vi "Format Data.vi"(0 "Potentiostat Galvanostat in":refnum<class "Potentiostat Galvanostat.lvclass">, 7 "Data Buffer":u32[][](array[numeric]), 11 "error in (no error)":errorcluster) -> (4 "Potentiostat Galvanostat out":refnum<class "Potentiostat Galvanostat.lvclass">, 8 "Data":sgl[][](array[numeric]), 15 "error out":errorcluster)   [LabVIEW 2018, in "Potentiostat Galvanostat.lvclass"]
doc: "The hardware conf object. The attribute “Conn” is the electrode\nconnection mode and the attribute “Ground” is the instrument\nground. See 5. Structures and Constants to have the value of these\nattributes."
uses:
  Potentiostat Galvanostat.lvclass
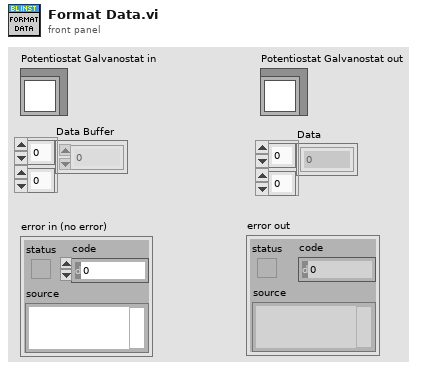
[diagram p1: front panel]
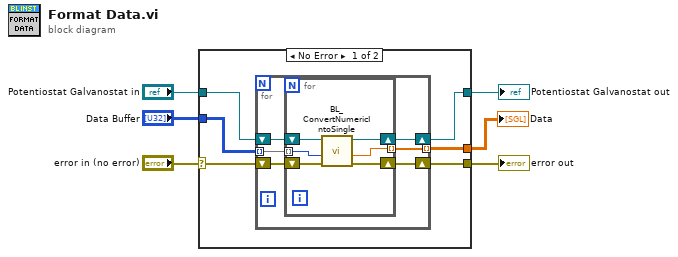
[diagram p0: block diagram]
diagram:
  n1 = case shown="No Error" "error in (no error)" {
    selector: "error in (no error)" -> [w8 w25]
    tunnel: "Data Buffer" -> [w7 _]
    tunnel: "Potentiostat Galvanostat in" -> [w12 w26]
    tunnel: [w11 _] -> w4
    tunnel: [w10 w25] -> w3
    tunnel: [w9 w26] -> w2
    frame No Error {
      n2 = for {
        tunnel: w7 -> [w18] mode=indexing
        tunnel: [w17] -> w11 mode=indexing
        shift-right: [w13] -> w10
        shift-left: w8 -> [w16]
        shift-right: [w14] -> w9
        shift-left: w12 -> [w15]
        n3 = for {
          tunnel: w18 -> [w24] mode=indexing
          tunnel: [w23] -> w17 mode=indexing
          shift-right: [w21] -> w13
          shift-left: w16 -> [w22]
          shift-right: [w19] -> w14
          shift-left: w15 -> [w20]
          n4 = call-dynamic "BL_ConvertNumericIntoSingle.vi"("error in (no error)"=w22, "Number"=w24, "Potentiostat Galvanostat in"=w20) -> ("error out"=w21:errorcluster, "Single"=w23:sgl, "Potentiostat Galvanostat out"=w19:refnum<class "Potentiostat Galvanostat.lvclass">)  [unwired: 6 in]
        }
      }
    }
    frame Error {
    }
  }
  "error out" <- w3
  "Potentiostat Galvanostat out" <- w2
  "Data" <- w4
